vi "Show or Hide QSettings.vi"(8 "error in (no error)":errorcluster, 11 "HIJ Vision Display in":refnum<class "HIJ Vision Display.lvclass">) -> (0 "error out":errorcluster, 3 "HIJ Vision Display out":refnum<class "HIJ Vision Display.lvclass">)   [LabVIEW 2014, in "HIJ Vision Display.lvlib" / "HIJ Vision Display.lvclass"]
uses:
  HIJ Vision Display.lvclass
  HIJ Vision Display.lvclass/HIJ Vision Display.ctl
  HIJ Vision Display Messages/Show or Hide Quick Settings Msg/Show or Hide Quick Settings Msg.lvclass/Show or Hide Quick Settings Msg.ctl
  <vilib>/ActorFramework/Message Enqueuer/Message Enqueuer.lvclass/Message Enqueuer.ctl
  <vilib>/ActorFramework/Message Enqueuer/Enqueue.vi
  <vilib>/ActorFramework/Message Priority Queue/Priority Enqueue.vi
  HIJ Vision Display Messages/Show or Hide Quick Settings Msg/Show or Hide Quick Settings Msg.lvclass
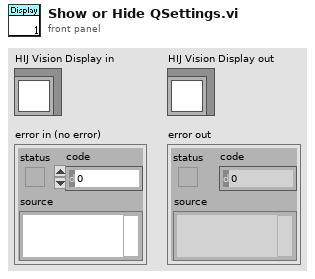
[diagram p1: front panel]
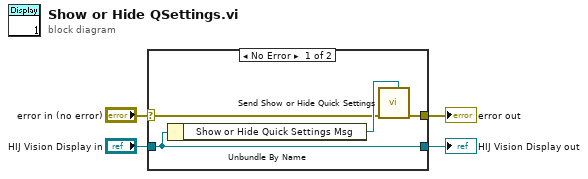
[diagram p0: block diagram]
diagram:
  n1 = case shown="No Error" "error in (no error)" {
    selector: "error in (no error)" -> [w6 w10]
    tunnel: [w5 w10] -> w3
    tunnel: [w8 w9] -> w1
    tunnel: "HIJ Vision Display in" -> [w8 w9]
    frame No Error {
      n2 = Unbundle By Name(w8) -> ("Show or Hide Quick Settings Msg"=w7:refnum<class "Show or Hide Quick Settings Msg.lvclass">)
      n3 = call "Send Show or Hide Quick Settings.vi"("Message Type"=w7, "error in (no error)"=w6) -> ("error out"=w5:errorcluster)  [unwired: 8 in, 1 out]
    }
    frame Error {
    }
  }
  "error out" <- w3
  "HIJ Vision Display out" <- w1
